vi "Target.vi"() -> ()   [LabVIEW 2025]
uses:
  <vilib>/Platform/TimedLoop/XDataNode/timing_clust.ctl
  <vilib>/Platform/TimedLoop/XDataNode/nitl_modes.ctl
  <vilib>/Platform/TimedLoop/XDataNode/wakeup.ctl
  <vilib>/rvi/Emulation/niFpgaSctlEmulationGetInTimedLoop.vi
  <vilib>/rvi/Emulation/niFpgaEmulationReportErrorSimple.vi
  <vilib>/rvi/Emulation/niFpgaGetClockAttributes.vi
  <vilib>/rvi/Emulation/niFpgaCriticalErrorInLSC.vi
  <vilib>/rvi/linearAlgebra/MatrixMultiply/simVIs/SubVI/nifxpla_MatrixMultiply_SimMatrixSizes.vi
  <vilib>/rvi/linearAlgebra/MatrixMultiply/simVIs/SubVI/nifxpla_MatrixMultiply_Sim4WireAdapterVector.vi
  <vilib>/rvi/linearAlgebra/MatrixMultiply/simVIs/SubVI/nifxpla_MatrixMultiply_SimFrameHandShake.vi
  <vilib>/rvi/linearAlgebra/MatrixMultiply/simVIs/SubVI/nifxpla_MatrixMultiply_SimEndlessCounter.vi
  <vilib>/rvi/linearAlgebra/MatrixMultiply/simVIs/SubVI/nifxpla_MatrixMultiply_SimVectorDataBuffer.vi
  <vilib>/rvi/ClientSDK/Core/DevComputerLib/Private/Multiply(dfxp64).vi
  <vilib>/rvi/ClientSDK/Core/DevComputerLib/Private/Dfxp128ToDfxp256.vi
  <vilib>/rvi/ClientSDK/Core/DevComputerLib/Private/Add(dfxp256).vi
  <vilib>/rvi/ClientSDK/Core/DevComputerLib/Private/Subtract(dfxp256).vi
  <vilib>/rvi/ClientSDK/Core/DevComputerLib/Private/ToDfxp64(dfxp256).vi
  <vilib>/platform/TimedLoop/XDataNode/XDataNode.xnode
  <vilib>/rvi/linearAlgebra/MatrixMultiply/XNode/nifxpla_MatrixMultiply.xnode
  <vilib>/rvi/linearAlgebra/MatrixMultiply/simVIs/nifxpla_MatrixMultiply_SimTemplateEinEout.vi
  <vilib>/rvi/linearAlgebra/MatrixMultiply/simVIs/nifxpla_MatrixMultiply_SimTemplateEinVout.vi
  <vilib>/rvi/linearAlgebra/MatrixMultiply/simVIs/nifxpla_MatrixMultiply_SimTemplateVinEout.vi
  <vilib>/rvi/linearAlgebra/MatrixMultiply/simVIs/nifxpla_MatrixMultiply_SimTemplateVinVout.vi
  <vilib>/Platform/TimedLoop/XDataNode/XDNodeRunTimeDep.lvlib
panel:
  out "C":fxp<+/-,32,16>[](array[numeric])
  out "Cycle Count":i32
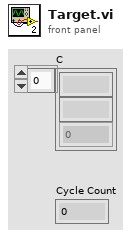
[diagram p1: front panel]
types:
  T1 = typedef "XDNodeRunTimeDep.lvlib/timing_clust.ctl" = cluster{"Expected End [f-1]":u64, "Actual End [f-1]":u64, "Finished Late? [f-1]":bool, "Expected End [i-1]":u64, "Actual End [i-1]":u64, "Finished Late? [i-1]":bool, "Expected Start [i]":u64, "Actual Start [i]":u64, "Expected Start [f]":u64, "Actual Start [f]":u64, "Source Name":string, "Structure Name":string, "Period":i64, "Deadline":i64, "Offset":i64, "Start":i64, "Priority":i32, "Timeout":i32, "Mode":T2, "Wakeup Reason":T3, "Error":errorcluster, "Source Type":string, "Secondary Source Type":string, "Global End Time":u64, "Global Start Time":u64, "Frame Duration":u64, "Iteration Duration":u64, "Assigned CPU":i32, "I/O Scan Engine Mode":u32}
  T2 = typedef "XDNodeRunTimeDep.lvlib/nitl_modes.ctl" = enum32{"No Change", "Process missed periods, maintain original phase", "Discard missed periods, maintain original phase", "Process missed periods, ignore original phase", "Discard missed periods, ignore original phase"}
  T3 = typedef "XDNodeRunTimeDep.lvlib/wakeup.ctl" = enum32{"Normal", "Aborted", "Asynchronous wakeup", "Timing source error", "Timed loop error", "Timeout"}
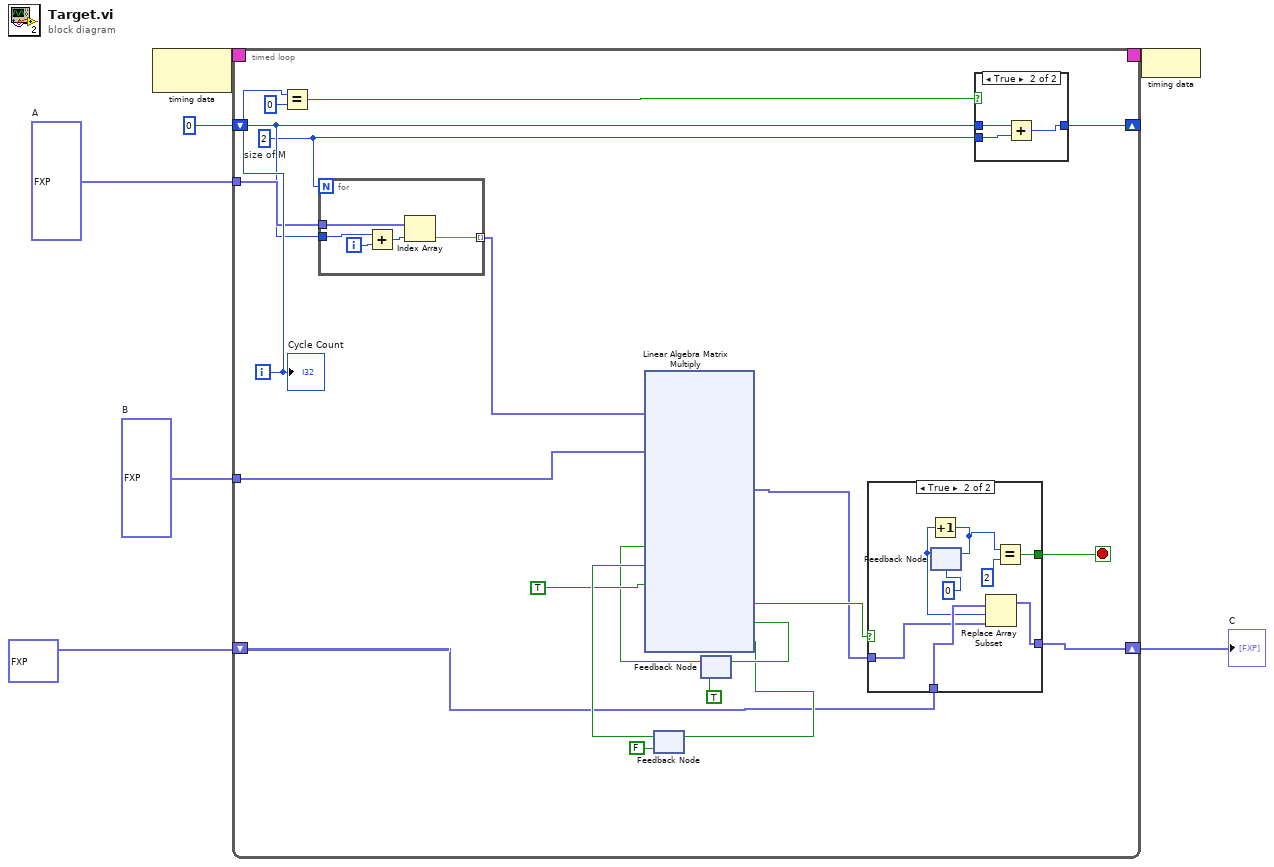
[diagram p0: block diagram]
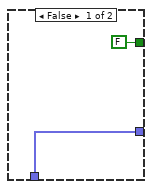
[diagram p3: hidden frame]
diagram:
  w3 = fxp<+/-,32,16>[] [1.0, 2.0, 3.0, 4.0]  # A
  w4 = fxp<+/-,32,16>[] [1.0, 2.0]  # B
  n1 = node-c288() -> (w7:T1)  [unwired: 1 in]
  n2 = timed-loop {
    timing: w7 -> [_]
    timing-out: [_] -> w6
    shift-right: [w20] -> w2
    shift-left: fxp<+/-,32,16>[] [0.0, 0.0] -> [w19]
    tunnel: w4 -> [w17]
    tunnel: w3 -> [w11]
    shift-right: [w13] -> _
    shift-left: 0 ("length") -> [w10]
    i -> [w15]
    stop <- w18 stop-if-true
    w8 = 2  # size of M
    n3 = Equal?(x=w15, y=0) -> (x = y?=w12:bool)
    n4 = for {
      N: w8 -> [_]
      tunnel: w11 -> [w33]
      tunnel: w10 -> [w31]
      tunnel: [w29] -> w9 mode=indexing
      i -> [w32]
      n5 = Add(x=w31, y=w32) -> (x+y=w30:i32)
      n6 = Index Array "Index Array"(array=w33, index=w30) -> (element=w29:fxp<+/-,32,16>)
    }
    n7 = feedback #1(FALSE ("ready for b")) -> (w26:bool)
    n8 = feedback #2(TRUE ("ready for a")) -> (w16:bool)
    n9 = xnode ("Linear Algebra Matrix Multiply")("ar"=w9, "br"=w17, "a valid"=w16, "b valid"=w26, "ready for output (T)"=TRUE) -> ("cr"=w21:fxp<+/-,32,16>[], "output valid"=w22:bool, "ready for a"=w28:bool, "ready for b"=w27:bool)  [unwired: 2 in, 2 out]
    n10 = feedback-in #1(w27) -> ()
    n11 = feedback-in #2(w28) -> ()
    n12 = case shown="True" w22 {
      tunnel: w21 -> [_ w42]
      tunnel: [w39 w46] -> w20
      tunnel: w19 -> [w39 w47]
      tunnel: [FALSE w43] -> w18
      frame False {
      }
      frame True {
        n13 = feedback #3(0 ("x")) -> (w41:i32)
        n14 = Increment(x=w41) -> (x+1=w40:i32)
        n15 = feedback-in #3(w40) -> ()
        n16 = Replace Array Subset(array=w47, new element=w42, index=w41) -> (w46:fxp<+/-,32,16>[])
        n17 = Equal?(x=w40, y=2) -> (x = y?=w43:bool)
      }
    }
    n18 = case shown="True" w12 {
      tunnel: w10 -> [w34 w37]
      tunnel: [w34 w36] -> w13
      tunnel: w8 -> [_ w35]
      frame False {
      }
      frame True {
        n19 = Add(x=w37, y=w35) -> (x+y=w36:i32)
      }
    }
    "Cycle Count" <- w15
  }
  "C" <- w2
  n20 = node-c288(w6) -> ()
